vi "Chroma 1905x Series Memory Get Location By Memory Name.vi"(7 "error in (no error)":errorcluster, 8 "Name":string, 10 "VISA resource name":refnum<visa-resource-name>) -> (0 "error out":errorcluster, 3 "VISA resource name out":refnum<visa-resource-name>, 9 "Memory Location":string)   [LabVIEW 2025]
doc: "Contact Chroma\nTEL: +886-2-2298-3855 \nTEL: +886-3-397-5788 \nFAX: +886-2-2298-3596\nFAX: +886-3-327-4703 \nURL: http://www.chromaate.com \nE-mail: chroma@chroma.com.tw"
panel:
  # "allowed characters: 0~9, A~Z, -"
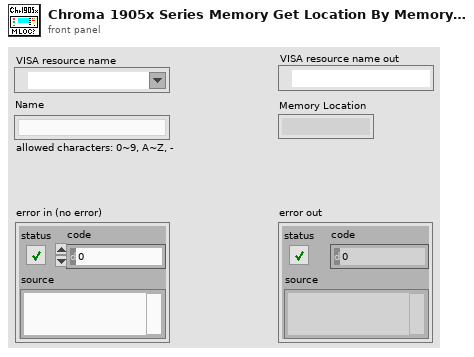
[diagram p1: front panel]
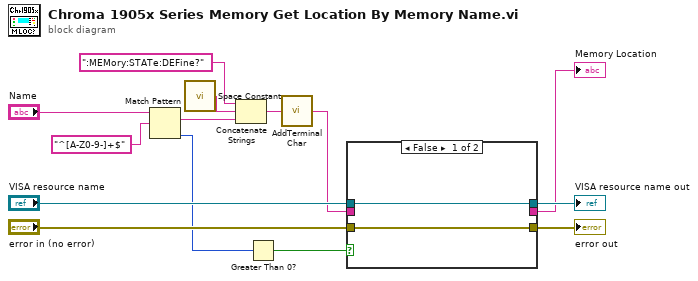
[diagram p0: block diagram]
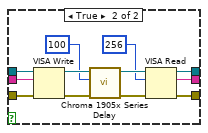
[diagram p2: hidden frame]
diagram:
  n1 = Match Pattern(string="Name", regular expression="^[A-Z0-9-]+$") -> (match substring=w4:string, offset past match=w7:i32)  [unwired: 1 in, 2 out]
  n2 = call <vilib>:"Space Constant.vi"() -> ("String"=w8:string)
  n3 = Concatenate Strings(":MEMory:STATe:DEFine?", w8, w4) -> (w1:string)
  n4 = Greater Than 0?(x=w7) -> (x > 0?=w3:bool)
  n5 = call "AddTerminal Char.vi"("Cmd string"=w1) -> ("Concatenated String"=w10:string)  [unwired: 4 in]
  n6 = case shown="False" w3 {
    tunnel: "error in (no error)" -> [w16 w24]
    tunnel: "VISA resource name" -> [w15 w22]
    tunnel: [w16 w23] -> w12
    tunnel: [w15 w21] -> w11
    tunnel: w10 -> [_ w17]
    tunnel: [_ w18] -> w2
    frame False {
    }
    frame True {
      n7 = VISA Write(VISA resource name=w22, write buffer=w17, error in (no error)=w24) -> (VISA resource name out=w27:refnum<visa-resource-name>, error out=w25:errorcluster)  [unwired: 1 out]
      n8 = call "Chroma 1905x Series Delay.vi"("error in (no error)"=w25, "Time Delay [ms]"=u32 100 ("Time Delay ms"), "VISA resource name"=w27) -> ("error out"=w26:errorcluster, "VISA resource name 2"=w28:refnum<visa-resource-name>)  [unwired: 7 in]
      n9 = VISA Read(VISA resource name=w28, byte count=u32 256, error in (no error)=w26) -> (VISA resource name out=w21:refnum<visa-resource-name>, read buffer=w18:string, error out=w23:errorcluster)  [unwired: 1 out]
    }
  }
  "error out" <- w12
  "VISA resource name out" <- w11
  "Memory Location" <- w2
